vi "Test_ConfigurationFileBinding_ValueOK.vi"(8 "error in (no error)":errorcluster, 11 "TestCase in":refnum<class "TestTransport.lvclass">) -> (0 "error out":errorcluster, 3 "TestCase out":refnum<class "TestTransport.lvclass">)   [LabVIEW 2015, in "Transport.lvlib" / "TestTransport.lvclass"]
uses:
  TestTransport.lvclass
  <vilib>/Utility/sysdir.llb/System Directory Type.ctl
  ConfigurationFileBinding/ConfigurationFileBinding.lvclass/ConfigurationFileBinding.ctl
  <vilib>/Utility/error.llb/Error Cluster From Error Code.vi
  <vilib>/Utility/config.llb/Not A Config Data Refnum.vi
  <vilib>/Utility/config.llb/Read Key (I32).vi
  ConfigurationFileBinding/ConfigurationFileBinding.lvclass
  <vilib>/Utility/config.llb/NI_LVConfig.lvlib
panel:
  out "Test File Path":path
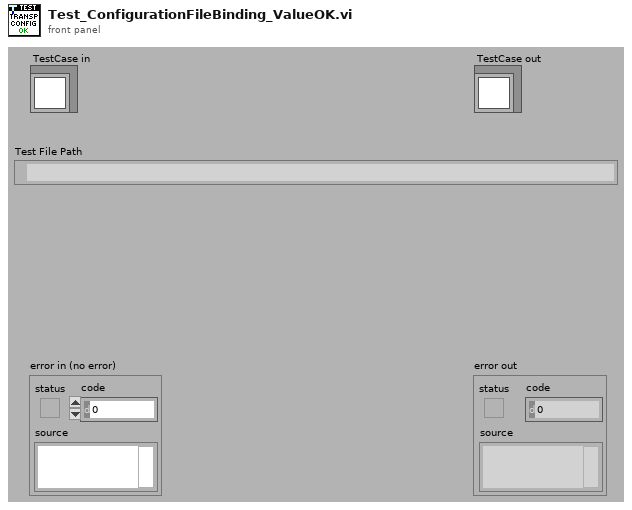
[diagram p1: front panel]
types:
  T1 = typedef "System Directory Type.ctl" = i32
  T2 = typedef "NI_LVConfig.lvlib/Config Data RefNum.ctl" = refnum<k1>
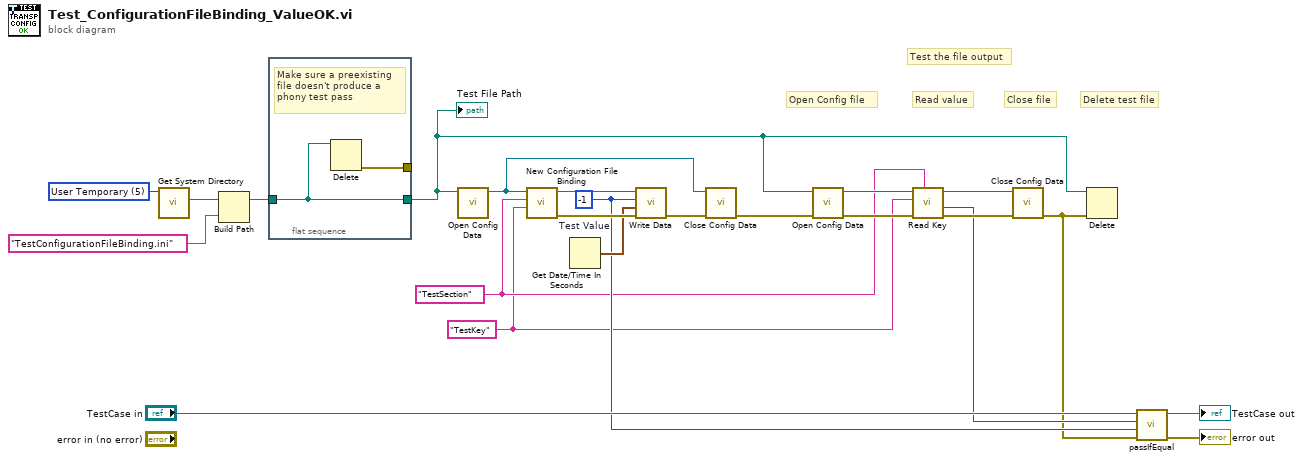
[diagram p0: block diagram]
diagram:
  w5 = "TestKey" ("Key Name")
  w6 = "TestSection" ("Section Name")
  w11 = -1  # Test Value
  w17 = T1 5 items=["User Home"=0, "User Desktop"=1, "User Documents"=2, "User Application Data"=3, "User Preferences"=4, "User Temporary"=5, "Public Documents"=6, "Public Application Data"=7, "Public Preferences"=8, "Public Cache"=13, "System Core Libraries"=9, "System Installed Libraries"=10, "Application Files"=11, "Boot Volume Root"=12] ("system directory type")
  # "Close file"
  # "Open Config file"
  # "Delete test file"
  # "Test the file output"
  # "Read value"
  n1 = call <vilib>:"Get System Directory.vi"("system directory type"=w17) -> ("system directory"=w16:path)  [unwired: 10 in]
  n2 = Build Path(base path=w16, name or relative path="TestConfigurationFileBinding.ini") -> (appended path=w12:path)
  n3 = flat-sequence {
    tunnel: w12 -> [w25]
    tunnel: [w25] -> w2
    tunnel: [w24] -> _
    frame #0 {
      # "Make sure a preexisting\nfile doesn't produce a\nphony test pass"
      n4 = Delete(path (use dialog)=w25) -> (error out=w24:errorcluster)  [unwired: 4 in, 2 out]
    }
  }
  n5 = call <vilib>:"Open Config Data.vi"("configuration file path"=w2) -> ("refnum"=w10:T2)  [unwired: 8 in, 2 out]
  n6 = call "New Configuration File Binding.vi"("Key Name"=w5, "Section Name"=w6, "Config File Refnum"=w10) -> ("error out"=w18:errorcluster, "ConfigurationFileBinding"=w19:refnum<class "ConfigurationFileBinding.lvclass">)  [unwired: 7 in]
  n7 = Get Date/Time In Seconds() -> (seconds since 1Jan1904=w13:timestamp)
  n8 = call-dynamic "Write Data.vi"("error in (no error)"=w18, "Publication Time"=w13, "Value"=w11, "ConfigurationFileBinding In"=w19) -> ("error out"=w14:errorcluster)  [unwired: 6 in, 1 out]
  n9 = call <vilib>:"Close Config Data.vi"("error in (no error)"=w14, "refnum"=w10) -> ("error out"=w8:errorcluster)  [unwired: 8 in, 1 out]
  n10 = call <vilib>:"Open Config Data.vi"("error in (no error)"=w8, "configuration file path"=w2) -> ("error out"=w23:errorcluster, "refnum"=w9:T2)  [unwired: 7 in, 1 out]
  n11 = call-poly <vilib>:"Read Key.vi"("section"=w6, "error in (no error)"=w23, "key"=w5, "refnum"=w9) -> ("error out"=w4:errorcluster, "value"=w3:i32, "refnum out"=w7:T2)  [unwired: 4 in, 1 out]
  n12 = call <vilib>:"Close Config Data.vi"("error in (no error)"=w4, "refnum"=w7) -> ("error out"=w1:errorcluster)  [unwired: 8 in, 1 out]
  n13 = Delete(path (use dialog)=w2, error in=w1) -> ()  [unwired: 3 in, 3 out]
  n14 = call-dynamic "passIfEqual.vi"("error in (no error)"=w1, "y"=w11, "x"=w3, "TestCase in"="TestCase in") -> ("error out"=→"error out":errorcluster, "TestCase out"=→"TestCase out":refnum<class "TestTransport.lvclass">)  [unwired: 6 in]
  "Test File Path" <- w2
